vi "PH_gentec_Powermeter.range 2 limit.vi"(1 "Range":T1 items=["Auto", "1 pJ", "3 pJ", "10 pJ", "30 pJ", "100 pJ", "300 pJ", "1 nJ", "3 nJ", "10 nJ", "30 nJ", "100 nJ", "300 nJ", "1 uJ", "3 uJ", "10 uJ", "30 uJ", "100 uJ", "300 uJ", "1 mJ", "3 mJ", "10 mJ", "30 mJ", "100 mJ", "300 mJ", "1 J", "3 J", "10 J", "30 J", "100 J", "300 J", "1 kJ", "3 kJ", "10 kJ", "30 kJ", "100 kJ", "300 kJ", "1 MJ", "3 MJ", "10 MJ", "30 MJ", "100 MJ", "300 MJ"]) -> (0 "limit":dbl)   [LabVIEW 2014, in "PH_gentec_Powermeter.lvlib"]
doc: "This VI calculates from the range chosen the upper energy value."
uses:
  PH_gentec_Powermeter.lvlib
  non_GPL/instr.lib/gentec-SOLO-PE/Driver/Type Defs/gentec-SOLO-PE.Scale.ctl
  non_GPL/instr.lib/gentec-SOLO-PE/gentec-SOLO-PE - Driver.lvlib
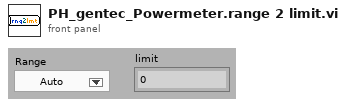
[diagram p1: front panel]
types:
  T1 = typedef "gentec-SOLO-PE - Driver.lvlib/gentec-SOLO-PE.Scale.ctl" = u32
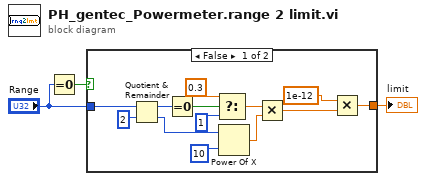
[diagram p0: block diagram]
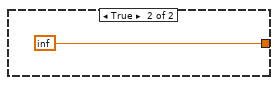
[diagram p2: hidden frame]
diagram:
  n1 = Equal To 0?(x="Range") -> (x = 0?=w2:bool)
  n2 = case shown="False" w2 {
    tunnel: [w4 inf] -> w3
    tunnel: "Range" -> [w12 _]
    frame False {
      n3 = Quotient & Remainder(x=w12, y=2) -> (x-y*floor(x/y)=w10:T1, floor(x/y)=w9:T1)
      n4 = Equal To 0?(x=w10) -> (x = 0?=w8:bool)
      n5 = Select(t=0.3 ("x/y"), s=w8, f=1) -> (s? t:f=w6:dbl)
      n6 = Power Of X(1:10 ("x"), 2:w9) -> (0:w15:dbl)
      n7 = Multiply(x=w6, y=w15) -> (x*y=w13:dbl)
      n8 = Multiply(x=1e-12, y=w13) -> (x*y=w4:dbl)
    }
    frame True {
    }
  }
  "limit" <- w3
